vi "TildaPassiveMain.vi"(0 "nOfBins":u32, 1 "delay_10ns_ticks":u32, 2 "TildaPassiveStateCtrl":T1) -> (20 "TildaPassiveStateInd":T1)   [LabVIEW 2014]
uses:
  Controls/TildaPassiveStates.ctl
  Controls/triggerTypes.ctl
  Controls/selectTrigger.ctl
  Controls/triggerEdge.ctl
  <vilib>/rvi/Emulation/niFpgaGetClockAttributes.vi
  <vilib>/rvi/Emulation/niFpgaSctlEmulationGetInTimedLoop.vi
  <vilib>/rvi/Emulation/niFpgaEmulationReportErrorSimple.vi
  <vilib>/rvi/Emulation/niFpgaCriticalErrorInLSC.vi
  <vilib>/rvi/Emulation/niFpgaProcessEmulError.vi
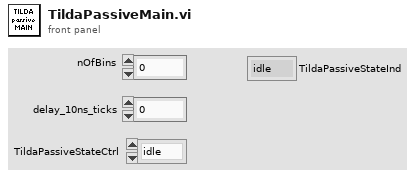
[diagram p1: front panel]
types:
  T1 = typedef "TildaPassiveStates.ctl" = enum16{"idle", "scanning", "error"}
  T2 = typedef "triggerEdge.ctl" = enum8{"either", "false-true", "true-false"}
  T3 = typedef "selectTrigger.ctl" = enum8{"Ext0", "Ext1", "Ext2", "Ext3", "Ext4", "Ext5", "Ext6", "Ext7", "Int0", "Int1", "Int2", "Int3", "Int4", "Int5", "Int6", "Int7"}
  T4 = typedef "triggerTypes.ctl" = enum16{"noTrigger", "singleHitDelay", "singleHit", "software", "sweep"}
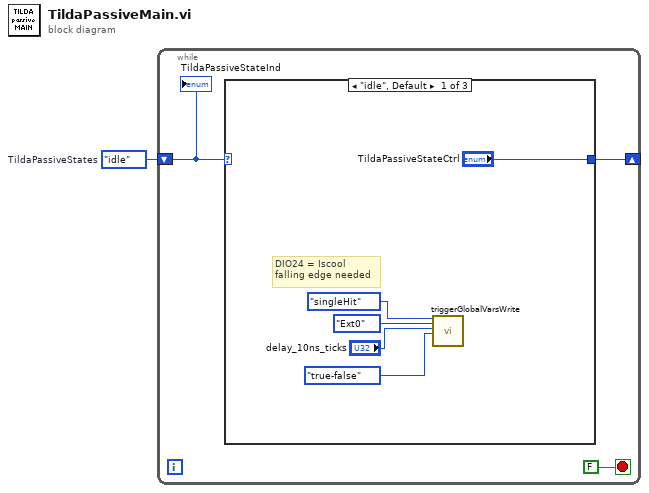
[diagram p0: block diagram]
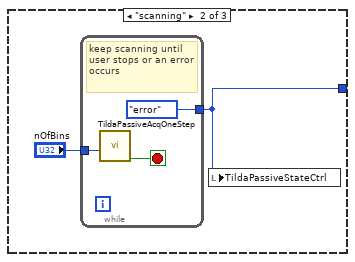
[diagram p2: hidden frame]
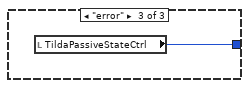
[diagram p3: hidden frame]
diagram:
  w1 = TildaPassiveStates."idle"  # TildaPassiveStates
  n1 = while {
    shift-right: [w2] -> _
    shift-left: w1 -> [w4]
    stop <- FALSE stop-if-true
    n2 = case shown="\"idle\", Default" w4 {
      tunnel: ["TildaPassiveStateCtrl" w10 w15] -> w2
      frame "idle", Default {
        # "DIO24 = Iscool\nfalling edge needed"
        n3 = call "triggerGlobalVarsWrite.vi"("triggerTypes"=triggerTypes."singleHit", "selectTrigger"=selectTrigger."Ext0", "delay_10ns_ticks"="delay_10ns_ticks", "triggerEdge"=triggerEdge."true-false") -> ()  [unwired: 16 in]
      }
      frame "scanning" {
        n4 = while {
          tunnel: "nOfBins" -> [w13]
          tunnel: [TildaPassiveStates."error" ("TildaPassiveStates")] -> w10
          stop <- w14 stop-if-true
          # "keep scanning until user stops or an error occurs"
          n5 = call "TildaPassiveAcqOneStep.vi"("nOfBins"=w13) -> ("abortOrTimeOut"=w14:bool)  [unwired: 10 in]
        }
        n6 = local write "TildaPassiveStateCtrl"(w10) -> ()
      }
      frame "error" {
        n7 = local read "TildaPassiveStateCtrl"() -> (w15:T1)
      }
    }
    "TildaPassiveStateInd" <- w4
  }
